vi "Main.vi"(11 "Module Admin":refnum<class "Delacor_lib_QMH_Cloneable Module Admin.lvclass">) -> ()   [LabVIEW 2022 SP3, in "HW-210_dqmh.lvlib"]
doc: "This template is based off of the Queued Message Handler design pattern and the Queued Message Handler project template that ships with LabVIEW.\n\nThe main difference is that the queue is private to this module and communication between modules is performed via Broadcast and Request events.\n\nRequest events are wrapped in public API methods and are handled in the Event Handling Loop (EHL) of this VI. Any module can register for Broadcast events sent by this module. The EHL generates messages based on user interface actions.\n\nThe Message Handling Loop (MHL) processes messages generated by the EHL, or by other messages. The messages are string values, so new messages can be added easily to the Message Cases case structure in the MHL. Each message cluster can also provide an optional value for Message Data, which is a variant that can be converted to whatever message-specific data is required.\n_____\nBased on DQMH Project Template 7.0.1.1316."
uses:
  HW-210_dqmh.lvlib
  <vilib>/Delacor/Delacor QMH/Libraries/Cloneable Module Admin_class/Delacor_lib_QMH_Cloneable Module Admin.lvclass
  C:/Program Files (x86)/National Instruments/LabVIEW 2022/vi.lib/Delacor/Delacor QMH/Libraries/Module Admin_class/Delacor_lib_QMH_Module Admin.lvclass
  Module Data--cluster.ctl
  <vilib>/Delacor/Delacor QMH/Libraries/Message Queue_class/Delacor_lib_QMH_Message Queue.lvclass/Delacor_lib_QMH_Message Queue.ctl
  <vilib>/Delacor/Delacor QMH/Libraries/Cloneable Module Admin_class/Delacor_lib_QMH_Cloneable Module Admin.lvclass/Delacor_lib_QMH_Cloneable Module Admin.ctl
  Stop Argument--cluster.ctl
  <vilib>/Delacor/Delacor QMH/Libraries/Module Admin_class/Delacor_lib_QMH_Module Admin.lvclass/Delacor_lib_QMH_Module Admin.ctl
  <vilib>/Utility/miscctls.llb/LVPointTypeDef.ctl
  <vilib>/Delacor/Delacor QMH/Libraries/Message Queue_class/Delacor_lib_QMH_Enqueue Message (Single).vi
  <vilib>/Delacor/Delacor QMH/Libraries/Cloneable Module Admin_class/Delacor_lib_QMH_Get Module ID.vi
  <vilib>/Delacor/Delacor QMH/Libraries/Module Admin_class/Delacor_lib_QMH_Get External Launch.vi
  <vilib>/Delacor/Delacor QMH/Libraries/Message Queue_class/Delacor_lib_QMH_Message Queue.lvclass
  <vilib>/MakerHub/LINX/Private/Device/Type Defs/Channels.ctl
  <vilib>/MakerHub/LINX/LMH-LINX.lvlib
  <vilib>/MakerHub/LINX/Private/Device/Type Defs/TCP Config.ctl
  <vilib>/MakerHub/LINX/Private/Device/Device.lvlib
  <vilib>/MakerHub/LINX/Private/Type Defs/Interface.ctl
  <vilib>/MakerHub/LINX/Private/Device/Type Defs/LINX Device Config.ctl
  <vilib>/MakerHub/LINX/Private/Type Defs/Platform.ctl
  <vilib>/MakerHub/LINX/Private/Type Defs/LINX Ref.ctl
  HW-201/HW-201.lvclass
  Motor/Motor.lvlib
panel:
  out "error out":errorcluster
  out "Status":string
  in  "Simulate EHL Error":bool
  in  "Simulate MHL Error":bool
  # "Other processes communicate with this Module via its Public API (wrappers for its Request Events).\n\nThis Module communicates with other processes via its Broadcast Events.\nAny process that wants to receive these messages can register for this module's Broadcast events."
  # "This template is for the DQMH framework. See the block diagram for more information on how to use this template."
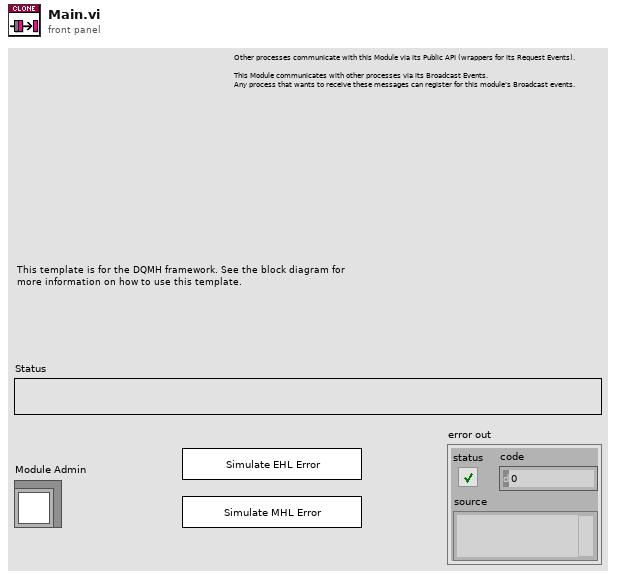
[diagram p1: front panel]
types:
  T1 = typedef "HW-210_dqmh.lvlib/Request Events--cluster.ctl" = cluster{"Stop Module":refnum<user-event>, "Show Panel":refnum<user-event>, "Hide Panel":refnum<user-event>, "Show Diagram":refnum<user-event>, "Get Module Execution Status":refnum<user-event>, "Linx Resource":refnum<user-event>}
  T2 = typedef "HW-210_dqmh.lvlib/Module Data--cluster.ctl" = cluster{"Status":string}
  T3 = typedef "LMH-LINX.lvlib/LINX Ref.ctl" = cluster{"IO":T4, "Interface":T5, "LINX Device Config":T6}
  T4 = typedef "LMH-LINX.lvlib/Platform.ctl" = enum16{"Remote", "Local"}
  T5 = typedef "LMH-LINX.lvlib/Interface.ctl" = enum16{"Serial", "TCP"}
  T6 = typedef "LMH-LINX.lvlib/Device.lvlib/LINX Device Config.ctl" = cluster{"Interface":T5, "COM Port":refnum<visa-resource-name>, "TCP Configuration":T7, "Device Family":u8, "Device ID":u8, "Device Name":string, "TCP Ref":refnum<k5>, "Channels":T8}
  T7 = typedef "LMH-LINX.lvlib/Device.lvlib/TCP Config.ctl" = cluster{"IP Address":string, "Port":u16}
  T8 = typedef "LMH-LINX.lvlib/Channels.ctl" = cluster{"DI":u8[], "DO":u8[], "AI":u8[], "AO":u8[], "PWM":u8[], "QE":u8[], "UART":u8[], "I2C 2":u8[], "SPI":u8[], "CAN":u8[], "Servo":u8[], "AI Ref (V)":dbl, "AI Resolution (Bits)":u8, "AO Ref (V)":dbl, "AO Resolution (Bits)":u8}
  T9 = enum32{"invalid lock state", "Not Locked", "Locked (No Password)", "Password-protected"}
  T10 = typedef "HW-210_dqmh.lvlib/Stop Argument--cluster.ctl" = cluster{"Module ID":i32, "Origin":string, "Exit via Stop Module Req?":bool, "Wait for Module to stop?":bool}
  T11 = typedef "LVPointTypeDef.ctl" = cluster{"Horizontal":i16, "Vertical":i16}
  T12 = enum32{"Invalid", "Standard", "Closed", "Hidden", "Minimized", "Maximized"}
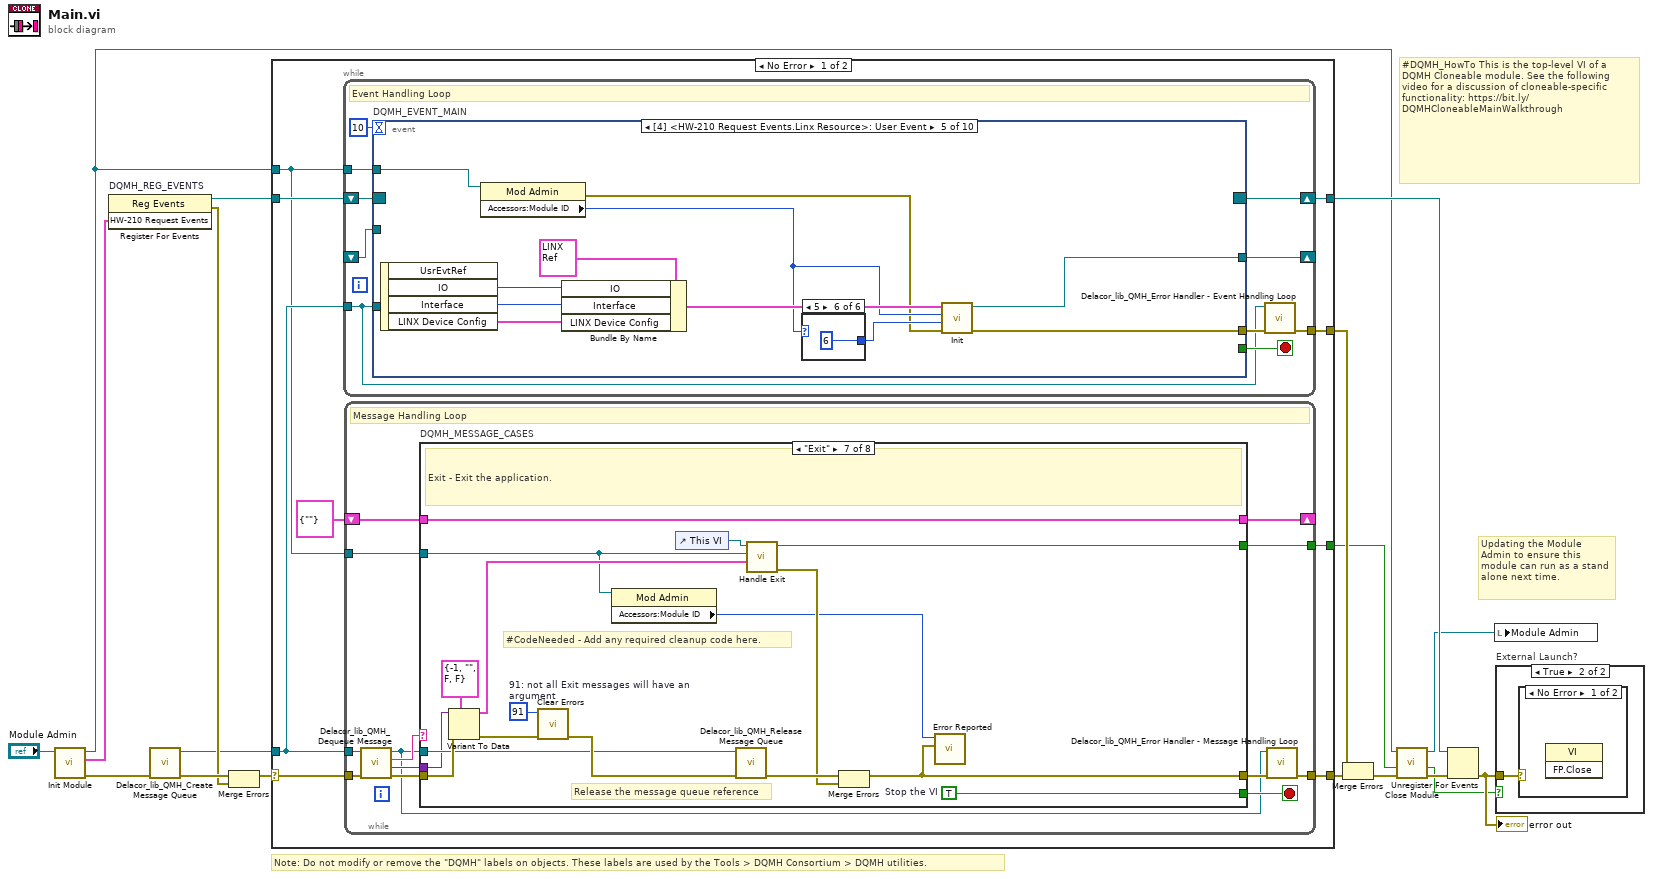
[diagram p0: block diagram]
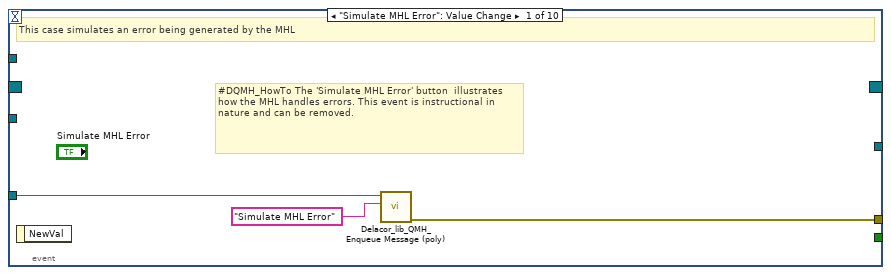
[diagram p2: hidden frame]
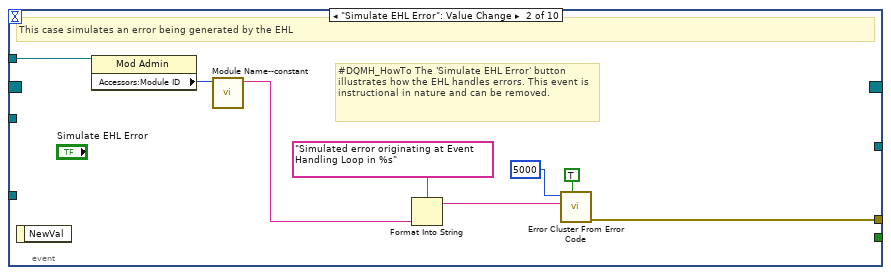
[diagram p3: hidden frame]
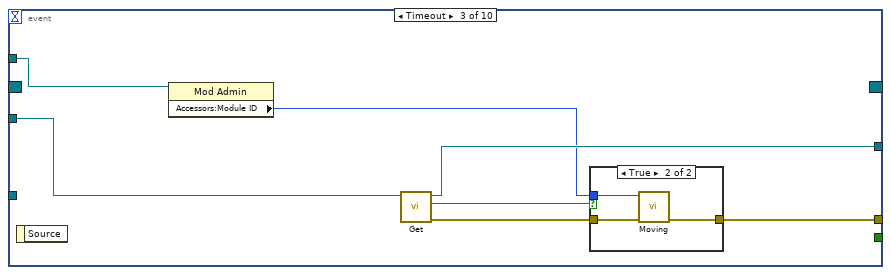
[diagram p4: hidden frame]
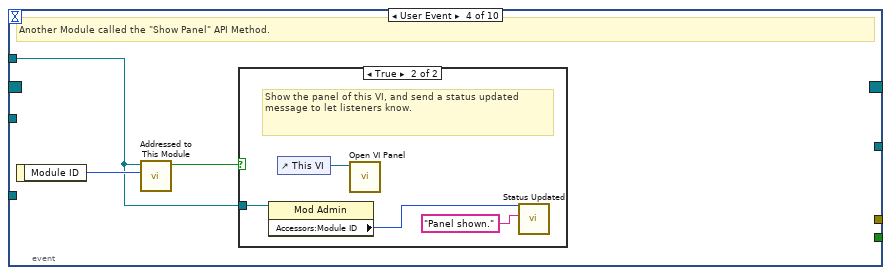
[diagram p6: hidden frame]
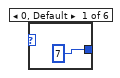
[diagram p8: hidden frame]
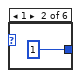
[diagram p9: hidden frame]
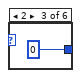
[diagram p10: hidden frame]
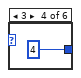
[diagram p11: hidden frame]
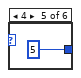
[diagram p12: hidden frame]
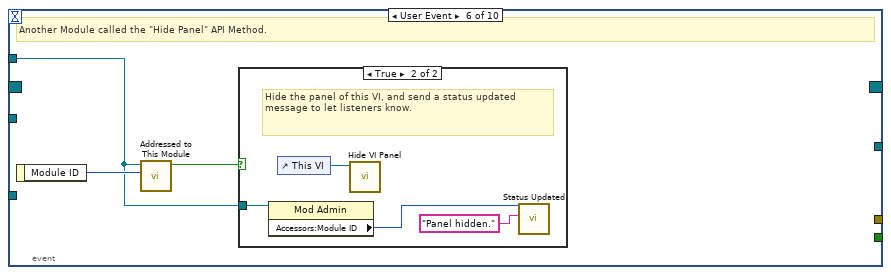
[diagram p13: hidden frame]
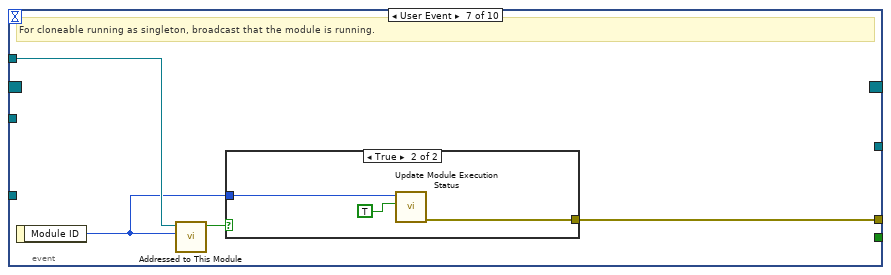
[diagram p15: hidden frame]
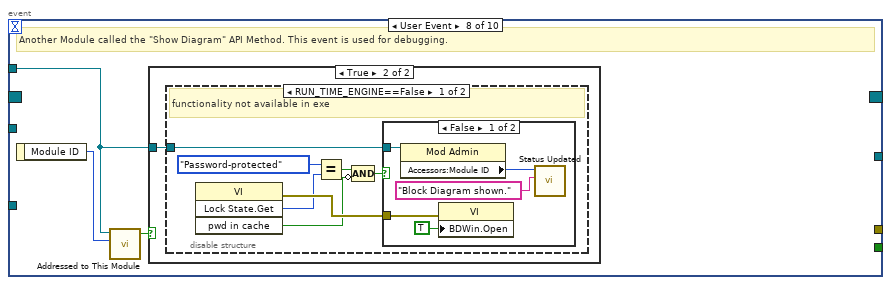
[diagram p17: hidden frame]
diagram:
  # "#DQMH_HowTo This is the top-level VI of a DQMH Cloneable module. See the following video for a discussion of cloneable-specific functionality: https://bit.ly/DQMHCloneableMainWalkthrough"
  # "Note: Do not modify or remove the \"DQMH\" labels on objects. These labels are used by the Tools > DQMH Consortium > DQMH utilities."
  # "Updating the Module Admin to ensure this module can run as a stand alone next time."
  n1 = call "Init Module.vi"("Cloneable Module Admin in"="Module Admin") -> ("error out"=w15:errorcluster, "HW-210 Request Events"=w7:T1, "Cloneable Module Admin out"=w4:refnum<class "Delacor_lib_QMH_Cloneable Module Admin.lvclass">)  [unwired: 8 in]
  n2 = register-events "DQMH_REG_EVENTS"(w7) -> (reference out=w8:refnum<event-registration>, error out=w10:errorcluster)  [unwired: 2 in]
  n3 = call <vilib>:"Delacor_lib_QMH_Create Message Queue.vi"("error in"=w15) -> ("error out"=w12:errorcluster, "Message Queue"=w6:refnum<class "Delacor_lib_QMH_Message Queue.lvclass">)  [unwired: 9 in]
  n4 = Merge Errors(w12, w10) -> (w11:errorcluster)
  n5 = case shown="No Error" w11 {
    selector: w11 -> [w25 w260]
    tunnel: [w27 w259] -> w16
    tunnel: [w24 w258] -> w9
    tunnel: w8 -> [w22 w258]
    tunnel: w6 -> [w21 w251]
    tunnel: [w26 _] -> w17
    tunnel: w4 -> [w20 w254]
    tunnel: [w19 _] -> w2
    frame No Error {
      n6 = while {
        tunnel: w21 -> [w31]
        shift-right: [w34] -> w24
        shift-left: w22 -> [w35]
        tunnel: [w36] -> w26
        tunnel: w20 -> [w32]
        shift-right: [w29] -> _
        shift-left: _ -> [w28]
        stop <- w33 stop-if-true
        # "Event Handling Loop"
        n7 = event "DQMH_EVENT_MAIN" shown="[4] <HW-210 Request Events.Linx Resource>: User Event" {
          selector: w35 -> [_ _ _ _ _ _ _ _ _ _]
          dyn-events: [_ _ _ _ _ _ _ _ _ _] -> w34
          timeout: 10 -> [_ _ _ _ _ _ _ _ _ _]
          tunnel: [_ _ _ _ _ _ _ _ w120 _] -> w33
          tunnel: w31 -> [w39 _ _ _ _ _ _ _ w123 w139]
          tunnel: [w40 w48 w52 _ w68 _ w94 _ w115 w142] -> w37
          tunnel: w32 -> [_ w47 w51 w60 w72 w84 w92 w98 w122 w140]
          tunnel: [_ _ w54 _ w67 _ _ _ _ _] -> w29
          tunnel: w28 -> [_ _ w55 _ _ _ _ _ w114 _]
          event "Simulate MHL Error": Value Change {
            # "#DQMH_HowTo The 'Simulate MHL Error' button  illustrates how the MHL handles errors. This event is instructional in nature and can be removed."
            # "This case simulates an error being generated by the MHL"
            n8 = event-data() -> ()  [unwired: 1 in, 1 out]
            n9 = call-poly <vilib>:"Delacor_lib_QMH_Enqueue Message (poly).vi"("Message"="Simulate MHL Error", "Message Queue in"=w39) -> ("error out"=w40:errorcluster)  [unwired: 8 in, 1 out]
          }
          event "Simulate EHL Error": Value Change {
            # "#DQMH_HowTo The 'Simulate EHL Error' button  illustrates how the EHL handles errors. This event is instructional in nature and can be removed."
            # "This case simulates an error being generated by the EHL"
            n10 = event-data() -> ()  [unwired: 1 in, 1 out]
            n11 = property on="Property Node" class="Mod Admin"(reference=w47) -> ("Accessors:Module ID"=w46:i32)  [unwired: 1 in, 2 out]
            n12 = call "Module Name--constant.vi"("Module ID"=w46) -> ("Module Name"=w41:string)  [unwired: 10 in]
            n13 = Format Into String(format string="Simulated error originating at Event Handling Loop in %s", w41) -> (resulting string=w44:string)  [unwired: 2 in, 1 out]
            n14 = call <vilib>:"Error Cluster From Error Code.vi"("show call chain? (False)"=TRUE, "error message (\"\")"=w44, "error code (0)"=5000) -> ("error out"=w48:errorcluster)  [unwired: 6 in]
          }
          event Timeout {
            n15 = event-data() -> ()  [unwired: 1 in, 1 out]
            n16 = property class="Mod Admin"(reference=w51) -> ("Accessors:Module ID"=w50:i32)  [unwired: 1 in, 2 out]
            n17 = call "Get.vi"("HW-201 in"=w55) -> ("error out"=w53:errorcluster, "isOnLine"=w49:bool, "HW-201 out"=w54:refnum<class "HW-201.lvclass">)  [unwired: 8 in]
            n18 = case shown="True" w49 {
              tunnel: w53 -> [w56 w59]
              tunnel: [w56 w58] -> w52
              tunnel: w50 -> [_ w57]
              frame False {
              }
              frame True {
                n19 = call "Moving.vi"("error in"=w59, "Modul"=w57) -> ("error out"=w58:errorcluster)  [unwired: 9 in]
              }
            }
          }
          event User Event {
            # "Another Module called the \"Show Panel\" API Method."
            n20 = event-data() -> ("Module ID"=w61:i32)  [unwired: 1 in]
            n21 = call "Addressed to This Module.vi"("Module ID from Argument"=w61, "Module Admin"=w60) -> ("Addressed to this instance?"=w62:bool)  [unwired: 8 in, 1 out]
            n22 = case shown="True" w62 {
              tunnel: w60 -> [_ w64]
              frame False {
              }
              frame True {
                # "Show the panel of this VI, and send a status updated message to let listeners know."
                n23 = property on="Property Node" class="Mod Admin"(reference=w64) -> ("Accessors:Module ID"=w63:i32)  [unwired: 1 in, 2 out]
                n24 = control-ref of="This VI"() -> (w66:refnum<vi>)
                n25 = call "Open VI Panel.vi"("VI"=w66) -> ()  [unwired: 10 in, 1 out]
                n26 = call "Status Updated.vi"("Status"="Panel shown." ("format string"), "Module ID"=w63) -> ()  [unwired: 9 in, 1 out]
              }
            }
          }
          event User Event {
            n27 = event-data() -> ("IO"=w76:T4, "Interface"=w75:T5, "LINX Device Config"=w74:T6)  [unwired: 1 in, 1 out]
            n28 = property class="Mod Admin"(reference=w72) -> (error out=w69:errorcluster, "Accessors:Module ID"=w71:i32)  [unwired: 1 in, 1 out]
            n29 = Bundle By Name(cluster=T3 {"IO"=enum."Remote", "Interface"=enum."Serial", "LINX Device Config"={"Interface"=enum."Serial", "COM Port"="", "TCP Configuration"={"IP Address"="", "Port"=0}, "Device Family"=0, "Device ID"=0, "Device Name"="", "TCP Ref"=refnum, "Channels"={"DI"=[], "DO"=[], "AI"=[], "AO"=[], "PWM"=[], "QE"=[], "UART"=[], "I2C 2"=[], "SPI"=[], "CAN"=[], "Servo"=[], "AI Ref (V)"=0.0, "AI Resolution (Bits)"=0, "AO Ref (V)"=0.0, "AO Resolution (Bits)"=0}}} ("LINX Resource"), "IO"=w76, "Interface"=w75, "LINX Device Config"=w74) -> (w73:T3)
            n30 = case shown="5" w71 {
              tunnel: [7 1 0 4 5 6] -> w70
              frame 0, Default {
              }
              frame 1 {
              }
              frame 2 {
              }
              frame 3 {
              }
              frame 4 {
              }
              frame 5 {
              }
            }
            n31 = call "Init.vi"("error in (no error)"=w69, "GPIO"=w70, "Number"=w71, "LINX Resource"=w73) -> ("error out"=w68:errorcluster, "HW-201 out"=w67:refnum<class "HW-201.lvclass">)  [unwired: 6 in]
          }
          event User Event {
            # "Another Module called the \"Hide Panel\" API Method."
            n32 = event-data() -> ("Module ID"=w85:i32)  [unwired: 1 in]
            n33 = call "Addressed to This Module.vi"("Module ID from Argument"=w85, "Module Admin"=w84) -> ("Addressed to this instance?"=w86:bool)  [unwired: 8 in, 1 out]
            n34 = case shown="True" w86 {
              tunnel: w84 -> [_ w88]
              frame False {
              }
              frame True {
                # "Hide the panel of this VI, and send a status updated message to let listeners know."
                n35 = property on="Property Node" class="Mod Admin"(reference=w88) -> ("Accessors:Module ID"=w87:i32)  [unwired: 1 in, 2 out]
                n36 = control-ref of="This VI"() -> (w90:refnum<vi>)
                n37 = call "Hide VI Panel.vi"("VI"=w90) -> ()  [unwired: 10 in, 1 out]
                n38 = call "Status Updated.vi"("Status"="Panel hidden." ("format string"), "Module ID"=w87) -> ()  [unwired: 9 in, 1 out]
              }
            }
          }
          event User Event {
            # "For cloneable running as singleton, broadcast that the module is running."
            n39 = event-data() -> ("Module ID"=w91:i32)  [unwired: 1 in]
            n40 = call "Addressed to This Module.vi"("Module ID from Argument"=w91, "Module Admin"=w92) -> ("Addressed to this instance?"=w93:bool)  [unwired: 8 in, 1 out]
            n41 = case shown="True" w93 {
              tunnel: [_ w97] -> w94
              tunnel: w91 -> [_ w96]
              frame False {
              }
              frame True {
                n42 = call "Update Module Execution Status.vi"("Running?"=TRUE, "Module ID"=w96) -> ("error out"=w97:errorcluster)  [unwired: 9 in]
              }
            }
          }
          event User Event {
            # "Another Module called the \"Show Diagram\" API Method. This event is used for debugging."
            n43 = event-data() -> ("Module ID"=w99:i32)  [unwired: 1 in]
            n44 = call "Addressed to This Module.vi"("Module ID from Argument"=w99, "Module Admin"=w98) -> ("Addressed to this instance?"=w100:bool)  [unwired: 8 in, 1 out]
            n45 = case shown="True" w100 {
              tunnel: w98 -> [_ w101]
              frame False {
              }
              frame True {
                n46 = disable-structure shown="RUN_TIME_ENGINE==False" {
                  disable-tunnel: w101 -> [w102 _]
                  frame condition #0 (active) {
                    # "functionality not available in exe"
                    n47 = invoke on="Invoke Node" class="VI" method="Lock State.Get"() -> (error out=w108:errorcluster, "Get Lock State"=w107:T9, "pwd in cache"=w104:bool)  [unwired: 4 in, 1 out]
                    n48 = Equal?(x=T9."Password-protected", y=w107) -> (x = y?=w105:bool)
                    n49 = Compound Arithmetic op=AND(w105, invert w104) -> (w103:bool)
                    n50 = case shown="False" w103 {
                      tunnel: w108 -> [w113 _]
                      tunnel: w102 -> [w110 _]
                      frame False {
                        n51 = property on="Property Node" class="Mod Admin"(reference=w110) -> ("Accessors:Module ID"=w109:i32)  [unwired: 1 in, 2 out]
                        n52 = property on="Property Node" class="VI"(error in=w113, "BDWin.Open"=TRUE ("Block Diagram Window:Open")) -> ()  [unwired: 1 in, 2 out]
                        n53 = call "Status Updated.vi"("Status"="Block Diagram shown." ("format string"), "Module ID"=w109) -> ()  [unwired: 9 in, 1 out]
                      }
                      frame True {
                        # "Password-protected VI, and the password is not in the cache. Do not show the diagram."
                      }
                    }
                  }
                  frame condition #1 {
                  }
                }
              }
            }
          }
          event User Event {
            # "Another Module called the \"Stop Module\" API Method  or the Message Handling Loop below."
            n54 = event-data() -> ("Module ID"=w118:i32, "Wait for Module to stop?"=w119:bool, "Origin"=w117:string)  [unwired: 1 in]
            n55 = call "Addressed to This Module.vi"("Module ID from Argument"=w118, "Module Admin"=w122) -> ("Addressed to this instance?"=w121:bool)  [unwired: 8 in, 1 out]
            n56 = case shown="True" w121 {
              tunnel: [_ w135] -> w116
              tunnel: w123 -> [_ w131]
              tunnel: [_ TRUE] -> w120
              tunnel: w119 -> [_ w126]
              tunnel: w118 -> [_ w128]
              tunnel: w117 -> [_ w124]
              frame False {
              }
              frame True {
                # "The event can get fired from the Exit message. The queue gets destroyed there. In this case, the Enqueue VI will return error 1. It is safe to ignore, because the module is already exiting."
                n57 = local write "Status"(w124) -> ()
                n58 = Bundle By Name(cluster=T10 {"Module ID"=-1, "Origin"="", "Exit via Stop Module Req?"=FALSE, "Wait for Module to stop?"=FALSE} ("Stop Argument"), "Module ID"=w128, "Exit via Stop Module Req?"=TRUE, "Wait for Module to stop?"=w126) -> (w125:T10)
                n59 = call-poly <vilib>:"Delacor_lib_QMH_Enqueue Message (poly).vi"("Priority Message? (F)"=TRUE, "Message Data"=w125, "Message"="Exit", "Message Queue in"=w131) -> ("error out"=w136:errorcluster)  [unwired: 6 in, 1 out]
                n60 = call <vilib>:"Clear Errors.vi"("error in (no error)"=w136, "specific error code to clear (0: all)"=1) -> ("error out"=w135:errorcluster)  [unwired: 4 in, 1 out]
              }
            }
            n61 = call "Close.vi"("error in (no error)"=w116, "HW-201 in"=w114) -> ("error out"=w115:errorcluster)  [unwired: 8 in, 1 out]
          }
          event Panel Close? {
            w141 = TRUE  # Discard the event, the MHL is responsible for closing and stopping this VI.
            # "Hide the panel or send the 'Exit' message if the user clicks the 'X' on the module main VI panel."
            n62 = event-data() -> ()  [unwired: 1 in, 1 out]
            n63 = property on="Property Node" class="Mod Admin"(reference=w140) -> (reference out=w137:refnum<class "Delacor_lib_QMH_Cloneable Module Admin.lvclass">, "Accessors:External Launch"=w138:bool)  [unwired: 1 in, 1 out]
            n64 = case shown="True" w138 {
              tunnel: w139 -> [_ w150]
              tunnel: [_ w151] -> w142
              tunnel: w137 -> [w145 _]
              frame True {
                # "If externally launched, clicking the 'X' hides the panel, but doesn't close it."
                n65 = property on="Property Node" class="Mod Admin"(reference=w145) -> ("Accessors:Module ID"=w144:i32)  [unwired: 1 in, 2 out]
                n66 = call "Status Updated.vi"("Status"="Panel hidden." ("format string"), "Module ID"=w144) -> ("error out"=w143:errorcluster)  [unwired: 9 in]
                n67 = control-ref of="This VI"() -> (w147:refnum<vi>)
                n68 = call "Hide VI Panel.vi"("error in"=w143, "VI"=w147) -> ()  [unwired: 9 in, 1 out]
              }
              frame False {
                # "If run as a stand-alone VI, clicking the panel 'X' stops the VI."
                n69 = call-poly <vilib>:"Delacor_lib_QMH_Enqueue Message (poly).vi"("Priority Message? (F)"=TRUE, "Message"="Exit", "Message Queue in"=w150) -> ("error out"=w151:errorcluster)  [unwired: 7 in, 1 out]
              }
            }
            n70 = event-data ("Event Filter Node")("Discard?"=w141) -> ()  [unwired: 1 in, 1 out]
          }
        }
        n71 = call-dynamic "Delacor_lib_QMH_Error Handler - Event Handling Loop.vi"("error in"=w37, "Message Queue in"=w31) -> ("dup error in"=w36:errorcluster)  [unwired: 8 in, 1 out]
      }
      n72 = while {
        tunnel: w21 -> [w152]
        shift-right: [w159] -> _
        shift-left: T2 {"Status"=""} ("Data Cluster") -> [w160]
        tunnel: w25 -> [w163]
        tunnel: [w161] -> w27
        tunnel: w20 -> [w154]
        tunnel: [w153] -> w19
        stop <- w158 stop-if-true
        # "Message Handling Loop"
        n73 = call-dynamic "Delacor_lib_QMH_Dequeue Message.vi"("error in"=w163, "Message Queue in"=w152) -> ("error out"=w162:errorcluster, "Message Data"=w156:variant, "Message"=w157:string, "Message Queue out"=w155:refnum<class "Delacor_lib_QMH_Message Queue.lvclass">)  [unwired: 6 in]
        n74 = case "DQMH_MESSAGE_CASES" shown="\"Exit\"" w157 {
          selector: w157 -> [_ _ _ _ _ _ _ w240]
          tunnel: w155 -> [_ _ _ _ w195 _ w232 _]
          tunnel: w162 -> [w183 w187 w190 w192 w204 w221 w238 w249]
          tunnel: [w181 w187 w189 w192 w200 w220 w233 w250] -> w164
          tunnel: w160 -> [w174 w186 w188 w191 w199 w218 w231 w247]
          tunnel: [w173 w186 w188 w191 w199 w218 w231 w247] -> w159
          tunnel: [_ _ _ _ _ _ w230 _] -> w158
          tunnel: w156 -> [_ _ _ _ w198 _ w228 _]
          tunnel: w154 -> [w168 _ _ _ w197 w216 w223 w246]
          tunnel: [_ _ _ _ _ _ w226 _] -> w153
          frame "Initialize" {
            w165 = "Initial Message" ("Initial Message")
            # "#CodeNeeded - Initialize the appearance of the front panel."
            # "#CodeNeeded - Initialize your state data here."
            # "Initialize - Any operation that needs to be done before the module can receive messages. Synchronize Caller Events.vi will inform Start Module.vi that the module has launched and is ready to receive messages. Module Did Init.vi will broadcast that the module initialized."
            n75 = call "Synchronize Caller Events.vi"("error in"=w183, "Module Admin"=w168) -> ("error out"=w182:errorcluster, "Module Admin out"=w167:refnum<class "Delacor_lib_QMH_Cloneable Module Admin.lvclass">)  [unwired: 8 in]
            n76 = property on="Property Node" class="Mod Admin"(reference=w167) -> ("Accessors:Module ID"=w170:i32, "Accessors:External Launch"=w169:bool)  [unwired: 1 in, 2 out]
            n77 = call "Module Name--constant.vi"("Module ID"=w170) -> ("Module Name"=w178:string)  [unwired: 10 in]
            n78 = property on="Property Node" class="VI"("Front Panel.Title"=w178) -> (reference out=w180:refnum<vi>, error out=w185:errorcluster)  [unwired: 2 in]
            n79 = Select(t=T12."Hidden" ("State"), s=w169, f=T12."Standard" ("State")) -> (s? t:f=w175:T12)
            n80 = invoke on="Invoke Node" class="VI" method="FP.Open"(reference=w180, error in=w185, "State"=w175) -> (reference out=w179:refnum<vi>, error out=w184:errorcluster)  [unwired: 2 in, 3 out]
            n81 = call "Module Name--constant.vi"("Module ID"=w170) -> ("Module Name"=w171:string)  [unwired: 10 in]
            n82 = Bundle By Name(cluster=w174, "Status"=w165) -> (w173:T2)
            n83 = invoke on="Invoke Node" class="VI" method="FP.Center"(reference=w179, error in=w184) -> ()  [unwired: 1 in, 3 out]
            n84 = property on="Pane" class="Pane"("Origin"=T11 {"Horizontal"=0, "Vertical"=0}) -> ()  [unwired: 2 in, 2 out]
            n85 = call "Module Did Init.vi"("error in"=w182, "Initialized?"=TRUE, "Origin"=w171, "Module ID"=w170) -> ("error out"=w181:errorcluster)  [unwired: 7 in]
            "Status" <- w165
          }
          frame "---Module Specific---" {
            # "Separator -- The following cases handle messages specific to this Module."
          }
          frame "---Copy This Frame---" {
            # "Duplicate this frame when creating new messages.  Change this comment in the duplicated frame to describe this message."
            n86 = Merge Errors(w190) -> (w189:errorcluster)
          }
          frame "---Exit and Error Handling---" {
            # "Separator - the following cases handle errors and exit messages."
          }
          frame "Error" {
            # "#CodeRecommended - If the module is running in standalone mode (External Launch = FALSE), this code will pop up an error dialog and call the 'Exit' message if an error occurs. Add more fine-grained error management here."
            # "Error - Check the error message data and respond accordingly. This message is sent by the \"Error Handler\" VIs at the end of each loop in this application."
            n87 = property on="Property Node" class="Mod Admin"(reference=w197) -> ("Accessors:External Launch"=w196:bool, "Accessors:Module ID"=w194:i32)  [unwired: 1 in, 2 out]
            n88 = Variant To Data(error in=w204, type=errorcluster {"status"=FALSE, "code"=0, "source"=""} ("error constant"), Variant=w198) -> (data=w193:errorcluster, error out=w202:errorcluster)
            n89 = local write "error out"(w193) -> ()
            n90 = call "Error Reported.vi"("Error"=w193, "Module ID"=w194) -> ()  [unwired: 9 in, 1 out]
            n91 = case shown="False" w196 {
              tunnel: [w209 _] -> w201
              tunnel: w195 -> [w207 _]
              tunnel: w193 -> [w208 _]
              frame False {
                n92 = disable-structure shown="Default" {
                  disable-tunnel: w208 -> [w210 _]
                  frame condition #0 (active) {
                    # "If the module is running standalone, then pop up an error dialog and call the \"Exit\" message."
                    n93 = call <vilib>:"Simple Error Handler.vi"("error in (no error)"=w210) -> ()  [unwired: 4 in, 5 out]
                  }
                  frame condition #1 {
                    # "To prevent the Simple Error Handler VI from being loaded (e.g. when deploying to a Real-Time target), add the Conditional Disable Symbol \"DQMH_Disable_SEH\" to your project and set it to TRUE."
                  }
                }
                n94 = call-poly <vilib>:"Delacor_lib_QMH_Enqueue Message (poly).vi"("Priority Message? (F)"=TRUE, "Message"="Exit", "Message Queue in"=w207) -> ("error out"=w209:errorcluster)  [unwired: 7 in, 1 out]
              }
              frame True {
                # "If the module was launched externally, calling the Error Reported broadcast VI is the only action performed by the \"Error\" message. The module's caller can then process the error appropriately."
              }
            }
            n95 = Merge Errors(w202, w201) -> (w200:errorcluster)
          }
          frame "Simulate MHL Error" {
            # "#DQMH_HowTo The 'Simulate MHL Error' button  illustrates how the MHL handles errors. This event is instructional in nature and can be removed."
            # "Simulate an error occurring at the MHL"
            n96 = property on="Property Node" class="Mod Admin"(reference=w216) -> ("Accessors:Module ID"=w217:i32)  [unwired: 1 in, 2 out]
            n97 = call "Module Name--constant.vi"("Module ID"=w217) -> ("Module Name"=w212:string)  [unwired: 10 in]
            n98 = Format Into String(format string="Simulated error originating at Message Handling Loop in %s", w212) -> (resulting string=w213:string)  [unwired: 2 in, 1 out]
            n99 = call <vilib>:"Error Cluster From Error Code.vi"("show call chain? (False)"=TRUE, "error message (\"\")"=w213, "error code (0)"=5001) -> ("error out"=w219:errorcluster)  [unwired: 6 in]
            n100 = Merge Errors(w221, w219) -> (w220:errorcluster)
          }
          frame "Exit" {
            w229 = 91  # 91: not all Exit messages will have an argument
            w230 = TRUE  # Stop the VI
            # "Release the message queue reference"
            # "#CodeNeeded - Add any required cleanup code here."
            # "Exit - Exit the application."
            n101 = Variant To Data(error in=w238, type=T10 {"Module ID"=-1, "Origin"="", "Exit via Stop Module Req?"=FALSE, "Wait for Module to stop?"=FALSE} ("Stop Argument"), Variant=w228) -> (data=w225:T10, error out=w234:errorcluster)
            n102 = call <vilib>:"Clear Errors.vi"("error in (no error)"=w234, "specific error code to clear (0: all)"=w229) -> ("error out"=w237:errorcluster)  [unwired: 4 in, 1 out]
            n103 = property on="Property Node" class="Mod Admin"(reference=w223) -> ("Accessors:Module ID"=w222:i32)  [unwired: 1 in, 2 out]
            n104 = control-ref of="This VI"() -> (w224:refnum<vi>)
            n105 = call-dynamic "Delacor_lib_QMH_Release Message Queue.vi"("error in"=w237, "Message Queue"=w232) -> ("error out"=w236:errorcluster)  [unwired: 9 in]
            n106 = call "Handle Exit.vi"("Stop Argument"=w225, "Module Admin in"=w223, "VI reference"=w224) -> ("error out"=w235:errorcluster, "Wait for Stop?"=w226:bool)  [unwired: 7 in]
            n107 = Merge Errors(w236, w235) -> (w233:errorcluster)
            n108 = call "Error Reported.vi"("Error"=w233, "Module ID"=w222) -> ()  [unwired: 9 in, 1 out]
          }
          frame Default {
            # "'Default' case only runs if there is a message that isn't defined in any of the other cases.  Output a programming error."
            n109 = property on="Property Node" class="Mod Admin"(reference=w246) -> ("Accessors:Module ID"=w245:i32)  [unwired: 1 in, 2 out]
            n110 = call "Module Name--constant.vi"("Module ID"=w245) -> ("Module Name"=w239:string)  [unwired: 10 in]
            n111 = Format Into String(format string="The invalid message string \"%s\" was received in the Message Handling Loop for module \"%s\".", w240, w239) -> (resulting string=w242:string)  [unwired: 2 in, 1 out]
            n112 = call <vilib>:"Error Cluster From Error Code.vi"("show call chain? (False)"=TRUE, "error message (\"\")"=w242, "error code (0)"=1) -> ("error out"=w248:errorcluster)  [unwired: 6 in]
            n113 = Merge Errors(w249, w248) -> (w250:errorcluster)
          }
        }
        n114 = call-dynamic "Delacor_lib_QMH_Error Handler - Message Handling Loop.vi"("error in"=w164, "Message Queue in"=w155) -> ("dup error in"=w161:errorcluster)  [unwired: 8 in, 1 out]
      }
    }
    frame Error {
      n115 = call "Synchronize Caller Events.vi"("Module Admin"=w254) -> ("Module Admin out"=w253:refnum<class "Delacor_lib_QMH_Cloneable Module Admin.lvclass">)  [unwired: 9 in, 1 out]
      n116 = property on="Property Node" class="Mod Admin"(reference=w253) -> ("Accessors:Module ID"=w252:i32)  [unwired: 1 in, 2 out]
      n117 = call-dynamic "Delacor_lib_QMH_Release Message Queue.vi"("error in"=w260, "Message Queue"=w251) -> ("error out"=w259:errorcluster)  [unwired: 9 in]
      n118 = call "Module Name--constant.vi"("Module ID"=w252) -> ("Module Name"=w257:string)  [unwired: 10 in]
      n119 = Format Into String(format string="An error occurred during initialization. %s is no longer running.", w257) -> (resulting string=w255:string)  [unwired: 2 in, 1 out]
      n120 = call "Error Reported.vi"("Additional Information"=w255, "Error"=w259, "Module ID"=w252) -> ()  [unwired: 8 in, 1 out]
    }
  }
  n121 = Merge Errors(w17, w16) -> (w18:errorcluster)
  n122 = call "Close Module.vi"("error in"=w18, "Wait for stop?"=w2, "Module Admin in"=w4) -> ("error out"=w14:errorcluster, "External Launch"=w1:bool, "Module Admin out"=w3:refnum<class "Delacor_lib_QMH_Cloneable Module Admin.lvclass">)  [unwired: 6 in]
  n123 = Unregister For Events(event registration refnum=w9, error in=w14) -> (error out=w13:errorcluster)
  "error out" <- w13
  n124 = local write "Module Admin"(w3) -> ()
  n125 = case "External Launch?" shown="True" w1 {
    tunnel: w13 -> [_ w261]
    frame False {
    }
    frame True {
      n126 = case shown="No Error" w261 {
        frame No Error {
          n127 = invoke class="VI" method="FP.Close"() -> ()  [unwired: 3 in, 3 out]
        }
        frame Error {
          n128 = invoke class="VI" method="FP.Open"("Activate"=TRUE ("Activate?")) -> ()  [unwired: 4 in, 5 out]
        }
      }
    }
  }
